vi "Get Channel Group Channels.vi"(8 "error in":errorcluster, 11 "channel group in":T1 format="%.0x") -> (0 "error out":errorcluster, 1 "channels":T1[](array[typedef]) format="%.0x", 2 "names":string[](array[string]), 3 "channel group out":T1 format="%.0x")   [LabVIEW 2027, in "Embedded Data Logger Scripting.lvlib"]
uses:
  Embedded Data Logger Scripting.lvlib
  <vilib>/NI VeriStand/Custom Device API/Custom Device Item Ref.ctl
  <vilib>/NI VeriStand/Custom Device API/Get Item Property (String Array).vi
  <vilib>/NI VeriStand/Custom Device API/Custom Device API.lvlib
  <vilib>/NI VeriStand/Custom Device Tools/Custom Device Utility Library/Custom Device Utility Library.lvlib
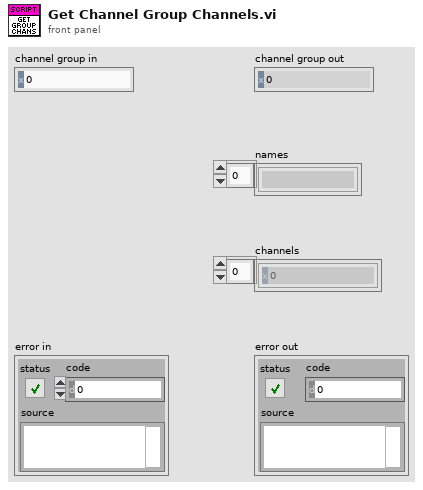
[diagram p1: front panel]
types:
  T1 = typedef "Custom Device API.lvlib/Custom Device Item Ref.ctl" = u64
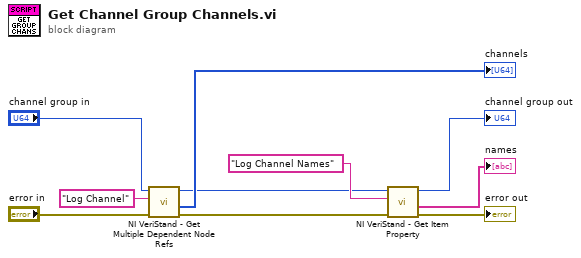
[diagram p0: block diagram]
diagram:
  n1 = call <vilib>:"NI VeriStand - Get Multiple Dependent Node Refs.vi"("error in (no error)"="error in", "Base Property Name"="Log Channel", "Item Ref in"="channel group in") -> ("error out"=w8:errorcluster, "Dependent Node Refs"=→"channels":T1[], "Item Ref out"=w2:T1)  [unwired: 6 in]
  n2 = call-poly <vilib>:"NI VeriStand - Get Item Property.vi"("error in (no error)"=w8, "Property Name"="Log Channel Names", "Item Ref in"=w2) -> ("error out"=→"error out":errorcluster, "Value"=→"names":string[], "Item Ref out"=→"channel group out":T1)  [unwired: 1 in, 5 out]
